vi "SPD.Save Measurments Result.vi"(6 "Temperature index":i32, 7 "Name":string="QE_", 8 "Error In":errorcluster, 9 "write to file":bool, 10 "Param index":i32=2, 11 "SPD.Stand Ctrl in":T1 {"spdDeviceSession"."hidSPD.Sturtup Values"."HV_bias" format="%#_6p, V"; "spdDeviceSession"."hidSPD.Sturtup Values"."TSet" format="%#_6p, DegC"; "spdDeviceSession"."hidSPD.Controller"."HV_bias" format="%#_6p, V"; "spdDeviceSession"."hidSPD.Controller"."TSet" format="%#_6p, DegC"}) -> (0 "Error Out":errorcluster, 3 "SPD.Stand Ctrl out":T1 {"spdDeviceSession"."hidSPD.Sturtup Values"."HV_bias" format="%#_6p, V"; "spdDeviceSession"."hidSPD.Sturtup Values"."TSet" format="%#_6p, DegC"; "spdDeviceSession"."hidSPD.Controller"."HV_bias" format="%#_6p, V"; "spdDeviceSession"."hidSPD.Controller"."TSet" format="%#_6p, DegC"})   [LabVIEW 2018]
uses:
  typedefs/SPD.Stand Ctrl.ctl
  Instruments/SPD HID Interface/hidSPDLibForLabView/LibVIs/hidSPD Controls/hidSPD Device Session.ctl
  Instruments/SPD HID Interface/hidSPDLibForLabView/LibVIs/hidSPD Controls/hidSPD Controller.ctl
  Instruments/SPD HID Interface/hidSPDLibForLabView/LibVIs/hidSPD Controls/hidSPD SPD Type.ctl
  Instruments/KC705 DevBoard/typedefs/DevB.Session.ctl
  Instruments/KeySight 53230A/typedefs/FreqC.Session.ctl
  Instruments/KeySight 8164B/KeySight 8164B LAN InstrLib/typedefs/KeySight 8164B control.ctl
  Instruments/LeCroy SDA830/typedefs/LeCroy.Session.ctl
  typedefs/SPD.Events.ctl
  ConfigFile/SPD.Config File ctrl.ctl
  <vilib>/Utility/config.llb/Config Data RefNum.ctl
  typedefs/SPD.Meas Result.ctl
  typedefs/SPD.Queues.ctl
  typedefs/SPD.Stand state.ctl
  Instruments/KeySight 8164B/KeySight 8164B LAN InstrLib.lvlib
  <vilib>/Utility/config.llb/NI_LVConfig.lvlib
  Instruments/SPD HID Interface/hidSPDLibForLabView/hidSPDLibForLabView.lvlib
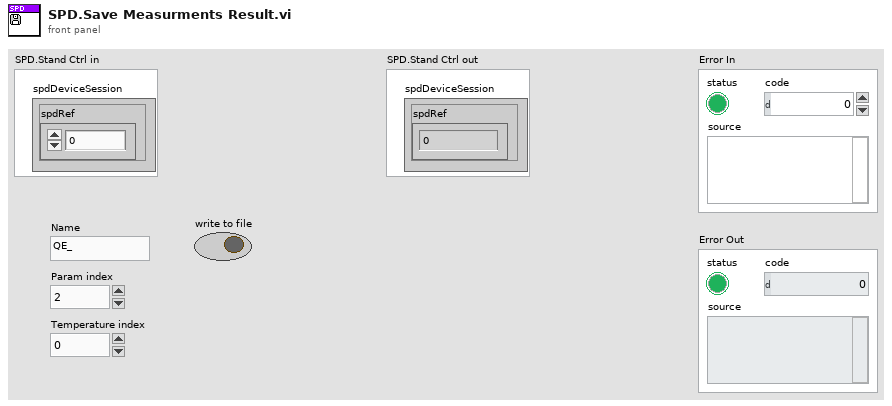
[diagram p1: front panel]
types:
  T1 = typedef "SPD.Stand Ctrl.ctl" = cluster{"spdDeviceSession":T2, "DevBSession":T5, "FreqCSession":T6, "8164BSession":T7, "LeCroySession":T8, "Events":T9, "configFile":T10, "SPD.Result":T12, "SPD.Queues":T13, "Console":refnum<vi>}
  T2 = typedef "hidSPDLibForLabView.lvlib/hidSPD Device Session.ctl" = cluster{"spdRef":u64, "connected":bool, "spdName":string, "hidSPD.Controller":T3, "hidSPD.Sturtup Values":T3, "SPD Type":T4}
  T3 = typedef "hidSPDLibForLabView.lvlib/hidSPD Controller.ctl" = cluster{"TSet":sgl, "HV_bias":sgl, "DDS_stb_code":u16}
  T4 = typedef "hidSPDLibForLabView.lvlib/hidSPD SPD Type.ctl" = enum16{"Free Run", "Gate"}
  T5 = typedef "DevB.Session.ctl" = cluster{"DevBRef":refnum<visa-resource-name>, "connected":bool}
  T6 = typedef "FreqC.Session.ctl" = cluster{"FreqCRef":refnum<visa-resource-name>, "timeout":dbl, "Gate":dbl, "connected":bool}
  T7 = typedef "KeySight 8164B LAN InstrLib.lvlib/KeySight 8164B control.ctl" = cluster{"Connection ID":refnum<k5>, "Connected":bool, "Info":string, "Slots Info":string[]}
  T8 = typedef "LeCroy.Session.ctl" = cluster{"LeCroySession":refnum<visa-resource-name>, "connected":bool}
  T9 = typedef "SPD.Events.ctl" = cluster{"DCRTest":refnum<user-event>, "Stop":refnum<user-event>}
  T10 = typedef "SPD.Config File ctrl.ctl" = cluster{"configFile ref":T11, "configFile path":path, "equipmentFile ref":T11}
  T11 = typedef "NI_LVConfig.lvlib/Config Data RefNum.ctl" = refnum<k1>
  T12 = typedef "SPD.Meas Result.ctl" = cluster{"HV_Bias":dbl[][][], "Stb_code":dbl[], "Temprature":dbl[], "Data":dbl[][][][], "DateTime":string}
  T13 = typedef "SPD.Queues.ctl" = cluster{"state queue":refnum<queue>}
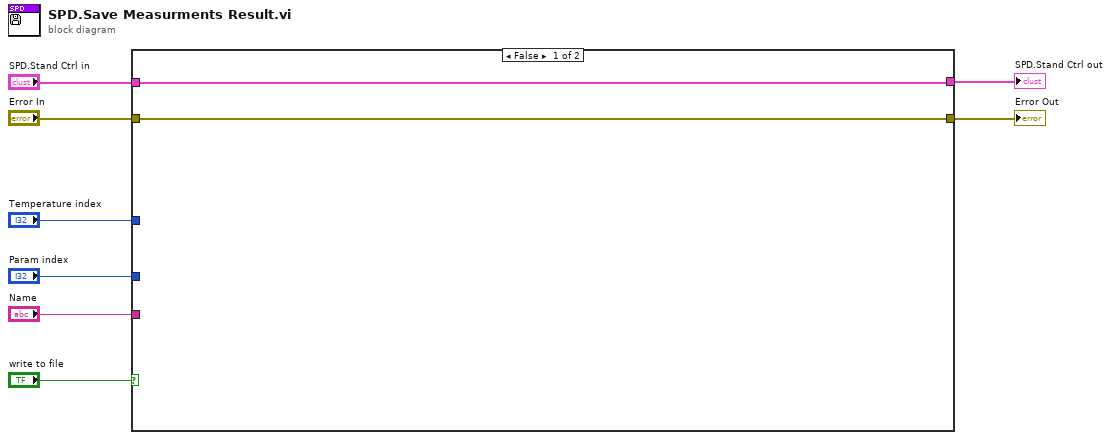
[diagram p0: block diagram]
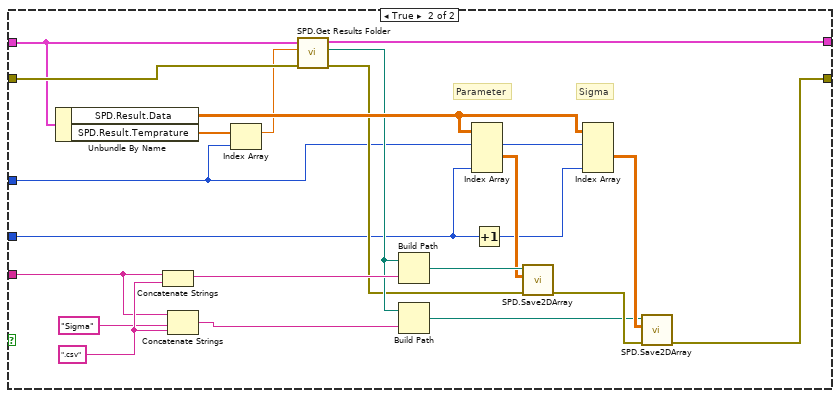
[diagram p2: hidden frame]
diagram:
  n1 = case shown="False" "write to file" {
    tunnel: [w9 w31] -> w8
    tunnel: "Error In" -> [w9 w30]
    tunnel: "SPD.Stand Ctrl in" -> [w10 w28]
    tunnel: [w10 w27] -> w5
    tunnel: "Name" -> [_ w22]
    tunnel: "Temperature index" -> [_ w13]
    tunnel: "Param index" -> [_ w12]
    frame False {
    }
    frame True {
      w25 = ".csv" ("string")
      # "Sigma"
      # "Parameter"
      n2 = Unbundle By Name(w28) -> ("SPD.Result.Data"=w32:dbl[][][][], "SPD.Result.Temprature"=w29:dbl[])
      n3 = Concatenate Strings(w22, w25) -> (w26:string)
      n4 = Concatenate Strings(w22, "Sigma", w25) -> (w23:string)
      n5 = Index Array(array=w29, index=w13) -> (element=w14:dbl)
      n6 = call "SPD.Get Results Folder.vi"("Error In"=w30, "Temperature"=w14, "SPD.Stand Ctrl in"=w28) -> ("Error Out"=w15:errorcluster, "Results path"=w16:path, "SPD.Stand Ctrl out"=w27:T1)  [unwired: 6 in]
      n7 = Build Path(base path=w16, name or relative path=w26) -> (appended path=w21:path)
      n8 = Build Path(base path=w16, name or relative path=w23) -> (appended path=w17:path)
      n9 = Index Array(array=w32, index (dim 0)=w13, index (dim 3)=w12) -> (element=w20:dbl[][])  [unwired: 2 in]
      n10 = Increment(x=w12) -> (x+1=w11:i32)
      n11 = call "SPD.Save2DArray.vi"("Error In"=w15, "Array"=w20, "File Path"=w21) -> ("Error Out"=w18:errorcluster)  [unwired: 8 in]
      n12 = Index Array(array=w32, index (dim 0)=w13, index (dim 3)=w11) -> (element=w19:dbl[][])  [unwired: 2 in]
      n13 = call "SPD.Save2DArray.vi"("Error In"=w18, "Array"=w19, "File Path"=w17) -> ("Error Out"=w31:errorcluster)  [unwired: 8 in]
    }
  }
  "SPD.Stand Ctrl out" <- w5
  "Error Out" <- w8
